vi "CANInit.vi"(8 "CAN1 Enable":bool, 11 "CAN Network Interface Config":T1={"Start On Open"=enum."TRUE", "Baud Rate"=500000, "Read Queue Length"=100, "Write Queue Length"=10, "Standard Comparator"=0, "Standard Mask"=0, "Extended Comparator"=0, "Extended Mask"=0} {"Baud Rate" min=5000 max=1333333 step=1; "Extended Mask" format="%.0x"; "Extended Comparator" format="%.0x"; "Standard Mask" format="%.0x"; "Standard Comparator" format="%.0x"; "Write Queue Length" max=1000; "Read Queue Length" max=1000}) -> (3 "Double CAN":T3)   [LabVIEW 2017]
uses:
  <vilib>/nican/nican.llb/xobjhandle.ctl
  <vilib>/nican/nican.llb/ncNetAttr.ctl
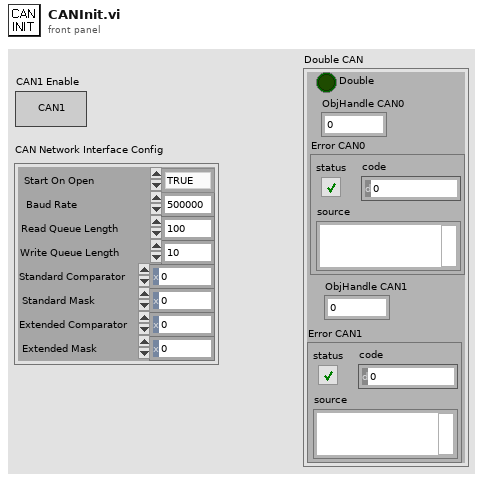
[diagram p1: front panel]
types:
  T1 = typedef "ncNetAttr.ctl" = cluster{"Start On Open":enum32{"FALSE", "TRUE"}, "Baud Rate":u32, "Read Queue Length":u32, "Write Queue Length":u32, "Standard Comparator":u32, "Standard Mask":u32, "Extended Comparator":u32, "Extended Mask":u32}
  T2 = typedef "xobjhandle.ctl" = u32
  T3 = cluster{"ObjHandle CAN0":T2, "Error CAN0":errorcluster, "Error CAN1":errorcluster, "ObjHandle CAN1":T2, "Double":bool}
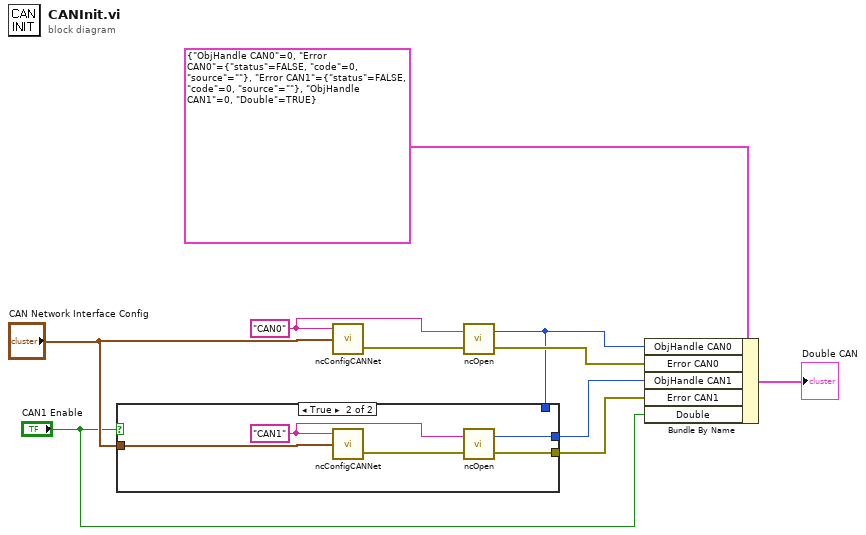
[diagram p0: block diagram]
diagram:
  w2 = "CAN0" ("ObjName")
  n1 = call <vilib>:"ncConfigCANNet.vi"("CAN Network Interface Config"="CAN Network Interface Config", "ObjName"=w2) -> ("Error out"=w3:errorcluster)  [unwired: 3 in]
  n2 = call <vilib>:"ncOpen.vi"("Error in"=w3, "ObjName"=w2) -> ("Error out"=w8:errorcluster, "ObjHandle out"=w4:T2)
  n3 = case shown="True" "CAN1 Enable" {
    tunnel: [w11 w14] -> w7
    tunnel: [_ w13] -> w6
    tunnel: "CAN Network Interface Config" -> [_ w12]
    tunnel: w4 -> [w11 _]
    frame False {
    }
    frame True {
      w16 = "CAN1" ("ObjName")
      n4 = call <vilib>:"ncConfigCANNet.vi"("CAN Network Interface Config"=w12, "ObjName"=w16) -> ("Error out"=w15:errorcluster)  [unwired: 3 in]
      n5 = call <vilib>:"ncOpen.vi"("Error in"=w15, "ObjName"=w16) -> ("Error out"=w13:errorcluster, "ObjHandle out"=w14:T2)
    }
  }
  n6 = Bundle By Name(cluster=T3 {"ObjHandle CAN0"=0, "Error CAN0"={"status"=FALSE, "code"=0, "source"=""}, "Error CAN1"={"status"=FALSE, "code"=0, "source"=""}, "ObjHandle CAN1"=0, "Double"=TRUE}, "ObjHandle CAN0"=w4, "Error CAN0"=w8, "ObjHandle CAN1"=w7, "Error CAN1"=w6, "Double"="CAN1 Enable") -> (→"Double CAN":T3)
